vi "Init scrollbar.vi"(7 "Scroll":refnum<vi>, 8 "error in (no error)":errorcluster caption="错误输入（无错误）", 10 "Data Len":i32, 11 "List":refnum<vi>) -> (0 "error out":errorcluster caption="错误输出", 3 "List out":refnum<vi>)   [LabVIEW 2018, in "CAN FD.lvlib"]
uses:
  CAN FD.lvlib
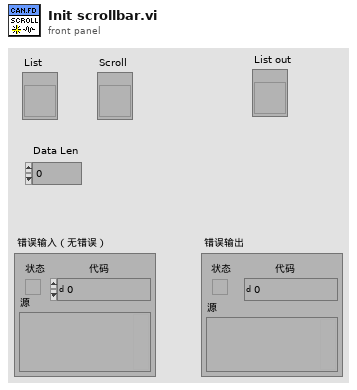
[diagram p1: front panel]
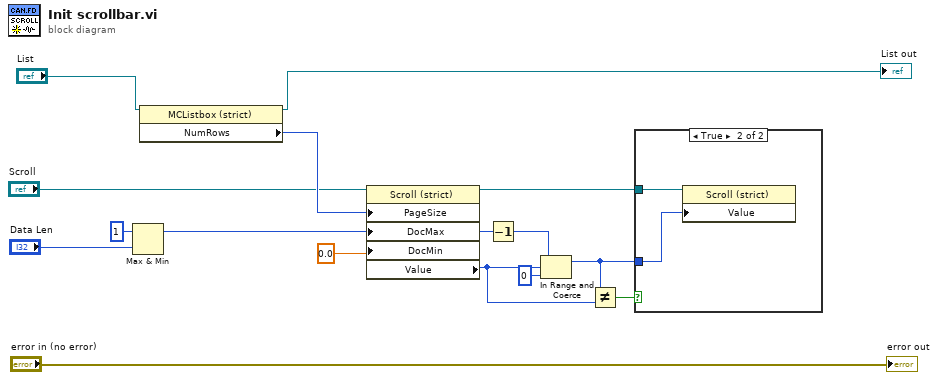
[diagram p0: block diagram]
diagram:
  n1 = Max & Min(x=1, y="Data Len") -> (max(x,y)=w1:i32)  [unwired: 1 out]
  n2 = property on="属性节点" class="MCListbox (strict)"(reference="List") -> (reference out=→"List out":refnum<vi>, "NumRows"=w15:u32)  [unwired: 1 in, 1 out]
  n3 = property on="属性节点" class="Scroll (strict)"(reference="Scroll", "PageSize"=w15, "DocMax"=w1, "DocMin"=0.0 ("滚动范围最小值")) -> (reference out=w3:refnum<vi>, "Value"=w5:i32)  [unwired: 1 in, 1 out]
  n4 = Decrement(x=w1) -> (x-1=w6:i32)
  n5 = In Range and Coerce(upper limit=w6, x=w5, lower limit=0 ("下限")) -> (coerced(x)=w2:i32)  [unwired: 1 out]
  n6 = Not Equal?(x=w2, y=w5) -> (x != y?=w4:bool)
  n7 = case shown="True" w4 {
    tunnel: w3 -> [_ w17]
    tunnel: w2 -> [_ w16]
    frame False {
    }
    frame True {
      n8 = property on="属性节点" class="Scroll (strict)"(reference=w17, "Value"=w16) -> ()  [unwired: 1 in, 2 out]
    }
  }
  "error out" <- "error in (no error)"
